vi "Test RP Lockin Scale.vi"() -> ()   [LabVIEW 2019]
panel:
  out "Slope":dbl=3.725290298461914e-09 format="%#_6p"
  in  "Range":dbl=1.0 format="%#_6eV"
  in  "Signal bits":i32=29
  in  "Decimation":u32=8192
  in  "Number of stages":i32=3
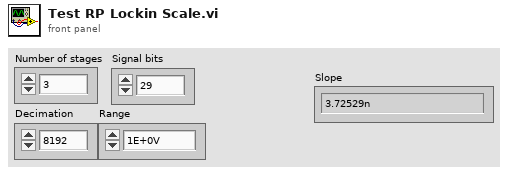
[diagram p1: front panel]
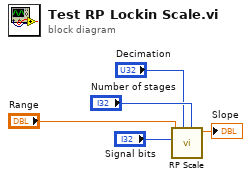
[diagram p0: block diagram]
diagram:
  n1 = call "RP Scale.vi"("Number of stages"="Number of stages", "Decimation"="Decimation", "Signal bits"="Signal bits", "Range"="Range") -> ("Slope"=→"Slope":dbl)  [unwired: 5 in, 2 out]
